vi "exec.vi"(8 "error in (no error)":errorcluster, 10 "context":refnum<class "IContextThisComponent.lvclass">, 11 "StopImageCapture in":refnum<class "StopImageCapture.lvclass">) -> (0 "error out":errorcluster, 2 "context 2":refnum<class "IContextThisComponent.lvclass">, 3 "StopImageCapture out":refnum<class "StopImageCapture.lvclass">)   [LabVIEW 2016, in "Commands.lvlib" / "StopImageCapture.lvclass"]
uses:
  StopImageCapture.lvclass
  IContextThisComponent/IContextThisComponent.lvclass
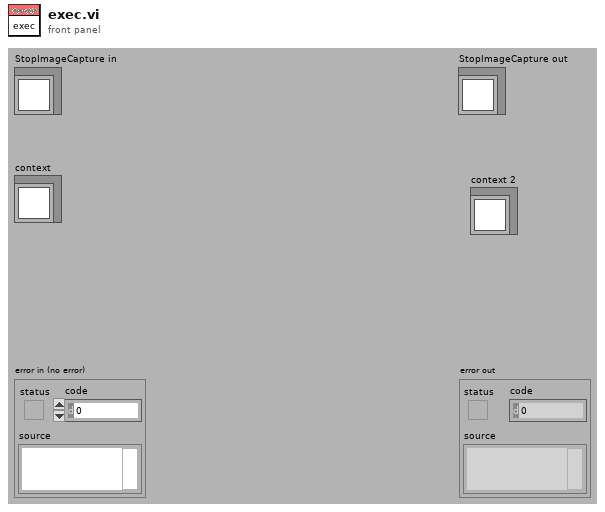
[diagram p1: front panel]
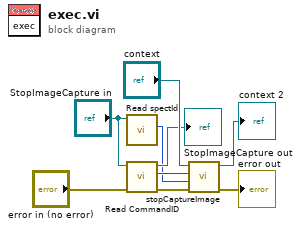
[diagram p0: block diagram]
diagram:
  n1 = call-dynamic "Read spectId.vi"("StopImageCapture in"="StopImageCapture in") -> ("spectId"=w1:u16)  [unwired: 8 in, 2 out]
  n2 = call-dynamic "Read CommandID.vi"("error in (no error)"="error in (no error)", "Command in"="StopImageCapture in") -> ("error out"=w5:errorcluster, "CommandID"=w4:i32, "Command out"=→"StopImageCapture out":refnum<class "StopImageCapture.lvclass">)  [unwired: 7 in]
  n3 = call-dynamic "stopCaptureImage.vi"("error in (no error)"=w5, "spectId"=w1, "CommandID"=w4, "IContextThisComponent in"="context") -> ("error out"=→"error out":errorcluster, "IContextThisComponent out"=→"context 2":refnum<class "IContextThisComponent.lvclass">)  [unwired: 6 in]
